vi "ExitAllReentrantVI.vi"(8 "error in (no error)":errorcluster, 11 "current queue name":string) -> (0 "error out":errorcluster)   [LabVIEW 2009]
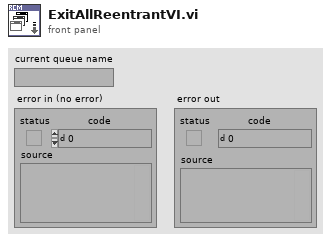
[diagram p1: front panel]
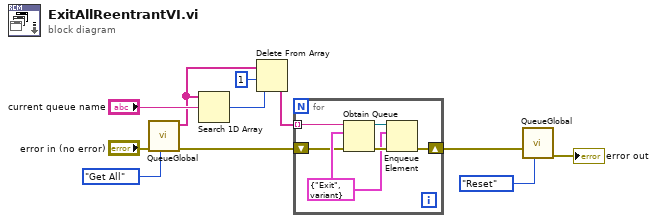
[diagram p0: block diagram]
diagram:
  n1 = call "QueueGlobal.vi"("cmd (Add)"=enum16{"Add One to End", "Get All", "Reset"}."Get All", "error in (no error)"="error in (no error)") -> ("error out"=w5:errorcluster, "queue names"=w9:string[])  [unwired: 8 in]
  n2 = Search 1D Array(1D array=w9, element="current queue name") -> (index of element=w8:i32)  [unwired: 1 in]
  n3 = Delete From Array(array=w9, length=1, index=w8) -> (array with subset deleted=w6:string[])  [unwired: 1 out]
  n4 = for {
    shift-right: [w17] -> w4
    shift-left: w5 -> [w12]
    tunnel: w6 -> [w13] mode=indexing
    w14 = cluster{"State":string, "Data":variant} {"State"="Exit", "Data"=variant} ("element")
    n5 = Obtain Queue(name (unnamed)=w13, element data type=w14, error in (no error)=w12) -> (queue out=w16:refnum<queue>, error out=w15:errorcluster)  [unwired: 2 in, 1 out]
    n6 = Enqueue Element(queue=w16, element=w14, error in (no error)=w15) -> (error out=w17:errorcluster)  [unwired: 1 in, 2 out]
  }
  n7 = call "QueueGlobal.vi"("cmd (Add)"=enum16{"Add One to End", "Get All", "Reset"}."Reset", "error in (no error)"=w4) -> ("error out"=→"error out":errorcluster)  [unwired: 8 in, 1 out]
